vi "LS370 Change Excitation act.vi"(0 "command text in":string[](array[string])) -> ()   [LabVIEW 2019]
uses:
  LS370 Excitation Voltage.ctl
  LS370 Resistance Range.ctl
panel:
  out "Mode":enum32{"Voltage", "Current"}(radio)
  out "VISA Resource Name":refnum<visa-resource-name> caption="VISA Name"
  out "Resistance Range":T1
  out "extra wait":i32 min=0
  out "Channel":i32=1 min=1 max=16 step=1
  out "Voltage":T2
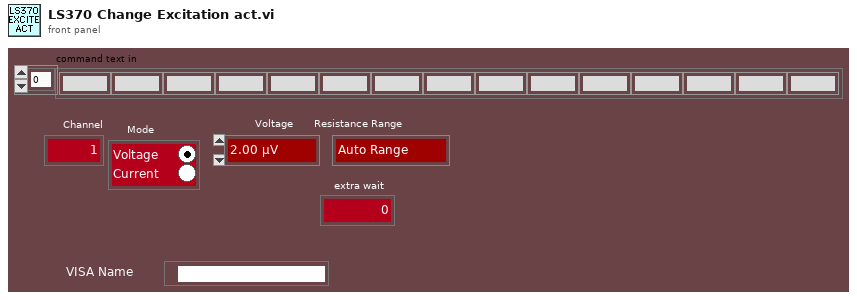
[diagram p1: front panel]
types:
  T1 = typedef "LS370 Resistance Range.ctl" = enum16{"Auto Range", "2.00 mΩ", "6.32 mΩ", "20.0 mΩ", "63.2 mΩ", "200 mΩ", "632 mΩ", "2.00 Ω", "6.32 Ω", "20.0 Ω", "63.2 Ω", "200 Ω", "632 Ω", "2.00 kΩ", "6.32 kΩ", "20.0 kΩ", "63.2 kΩ", "200 kΩ", "632 kΩ", "2.00 MΩ", "6.32 MΩ", "20.0 MΩ", "63.2 MΩ"}
  T2 = typedef "LS370 Excitation Voltage.ctl" = enum16{"2.00 µV", "6.32 µV", "20.0 µV", "63.2 µV", "200 µV", "632 µV", "2.00 mV", "6.32 mV", "20.0 mV", "63.2 mV", "200 mV", "632 mV"}
  T3 = enum16{"Auto Range", "2.00 m½", "6.32 m½", "20.0 m½", "63.2 m½", "200 m½", "632 m½", "2.00 ½", "6.32 ½", "20.0 ½", "63.2 ½", "200 ½", "632 ½", "2.00 k½", "6.32 k½", "20.0 k½", "63.2 k½", "200 k½", "632 k½", "2.00 M½", "6.32 M½", "20.0 M½", "63.2 M½"}
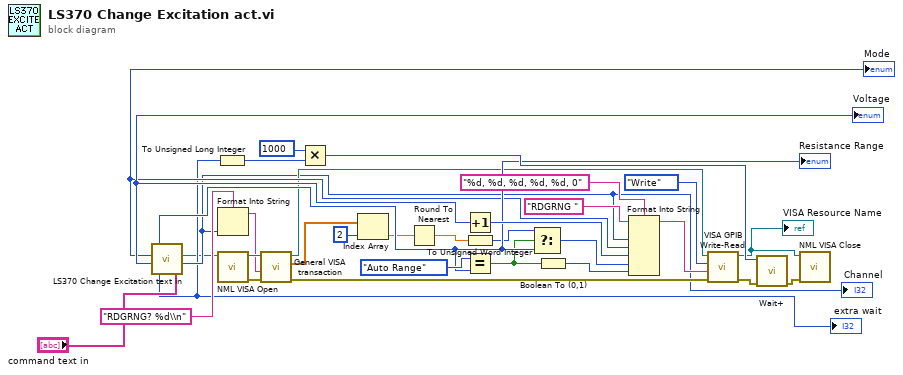
[diagram p0: block diagram]
diagram:
  n1 = call "LS370 Change Excitation text in.vi"("command text in"="command text in") -> ("Channel"=w5:i32, "VISA Refnum in"=w2:refnum<visa-resource-name>, "extra wait"=w4:i32, "Current"=w20:u16, "Mode"=w19:enum32{"Voltage", "Current"}, "Resistance Range"=w21:T1)  [unwired: 1 out]
  "Voltage" <- w20
  "Channel" <- w5
  "extra wait" <- w4
  "Resistance Range" <- w21
  "Mode" <- w19
  n2 = To Unsigned Long Integer(number=w4) -> (unsigned 32bit integer=w32:u32)
  n3 = Format Into String(format string="RDGRNG? %d\\n" ("Command String"), w5) -> (resulting string=w3:string)  [unwired: 2 in, 1 out]
  n4 = call "NML VISA Open.vi"("VISA resource name"=w2) -> ("error out"=w9:errorcluster, "VISA resource name out"=w10:refnum<visa-resource-name>)  [unwired: 9 in]
  n5 = call "General VISA transaction.vi"("error in (no error)"=w9, "Command String"=w3, "VISA Session"=w10) -> ("error out"=w8:errorcluster, "Measurement"=w15:dbl[], "dup VISA Session"=w16:refnum<visa-resource-name>)  [unwired: 3 in, 3 out]
  n6 = Multiply(x=u32 1000 ("y"), y=w32) -> (x*y=w31:u32)
  n7 = Index Array(array=w15, index=2) -> (element=w13:dbl)
  n8 = Round To Nearest(number=w13) -> (nearest integer value=w12:dbl)
  n9 = Increment(x=w20) -> (x+1=w27:u16)
  n10 = To Unsigned Word Integer(number=w12) -> (unsigned 16bit integer=w11:u16)
  n11 = Equal?(x=T3."Auto Range" ("y"), y=w21) -> (x = y?=w17:bool)
  n12 = Select(t=w11, s=w17, f=w21) -> (s? t:f=w25:u16)
  n13 = Boolean To (0,1)(Boolean=w17) -> (0, 1=w24:i16)
  n14 = Format Into String(format string="%d, %d, %d, %d, %d, 0", initial string="RDGRNG ", w5, w19, w27, w25, w24) -> (resulting string=w23:string)  [unwired: 1 in, 1 out]
  n15 = call "VISA GPIB Write-Read.vi"("error in (no error)"=w8, "Command"=w23, "Action"=enum16{"Write", "Read", "Write & Read"}."Write", "VISA resource name"=w16) -> ("error out"=w30:errorcluster, "dup VISA Session"=w1:refnum<visa-resource-name>)  [unwired: 4 in, 2 out]
  "VISA Resource Name" <- w1
  n16 = call "Wait+.vi"("Error In"=w30, "milliseconds to wait"=w31) -> ("Error Out"=w7:errorcluster)  [unwired: 4 in, 1 out]
  n17 = call "NML VISA Close.vi"("Error In"=w7, "VISA resource name"=w1) -> ()  [unwired: 9 in, 1 out]
